vi "PXI-Change AO Gains (gracefully).vi"(0 "Multipliers in":dbl[](array[numeric]), 5 "Gains":dbl[](array[numeric]), 11 "error in (no error)":errorcluster) -> (15 "error out":errorcluster)   [LabVIEW 2015]
uses:
  PXI Globals.vi
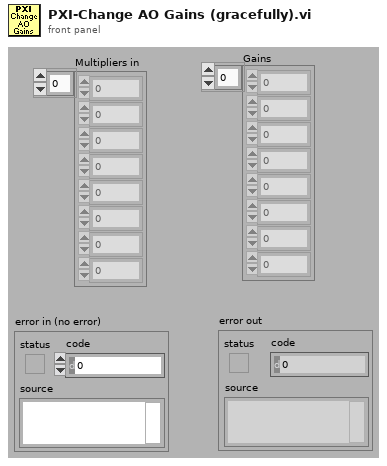
[diagram p1: front panel]
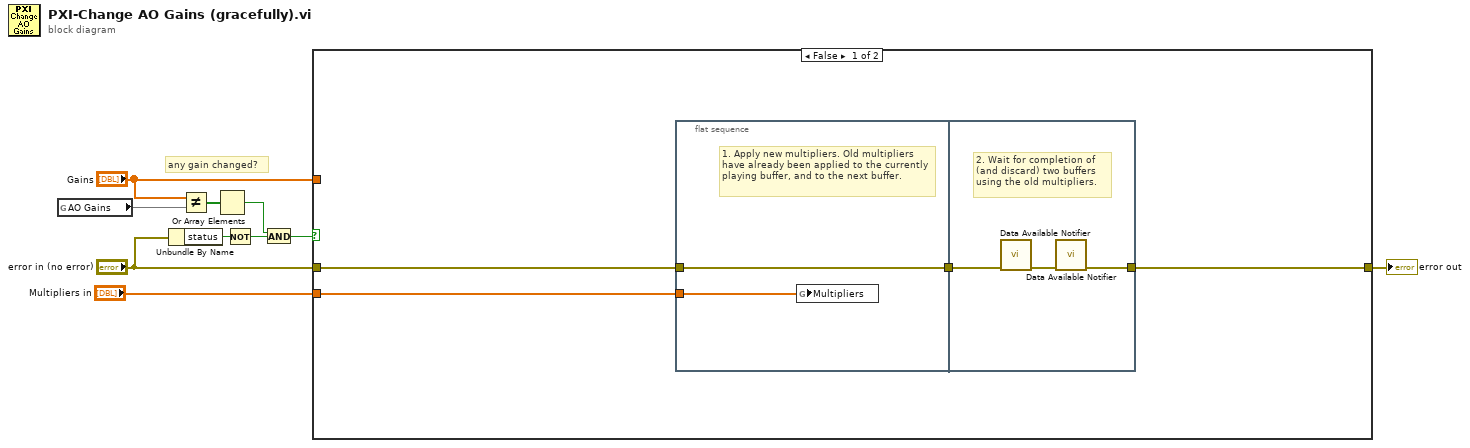
[diagram p0: block diagram]
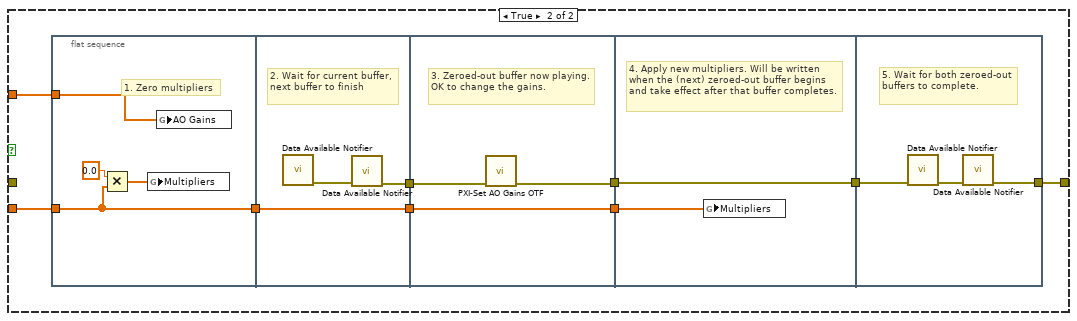
[diagram p2: hidden frame]
diagram:
  # "any gain changed?"
  n1 = global read "PXI Globals.vi" "AO Gains"() -> (w10)
  n2 = Unbundle By Name("error in (no error)") -> ("status"=w9:bool)
  n3 = Not Equal?(x="Gains", y=w10) -> (x != y?=w6:bool[])
  n4 = Or Array Elements(Boolean array=w6) -> (logical OR=w5:bool)
  n5 = Not(x=w9) -> (.not. x?=w8:bool)
  n6 = And(x=w5, y=w8) -> (x .and. y?=w7:bool)
  n7 = case shown="False" w7 {
    tunnel: "error in (no error)" -> [w12 _]
    tunnel: [w11 w28] -> w3
    tunnel: "Multipliers in" -> [w13 w27]
    tunnel: "Gains" -> [_ w20]
    frame False {
      n8 = flat-sequence {
        tunnel: [w15] -> w14
        tunnel: w13 -> [w16]
        tunnel: w12 -> [w15]
        tunnel: [w17] -> w11
        tunnel: w14 -> [w19]
        frame #0 {
          # "1. Apply new multipliers. Old multipliers have already been applied to the currently playing buffer, and to the next buffer."
          n9 = global write "PXI Globals.vi" "Multipliers"(w16) -> ()
        }
        frame #1 {
          # "2. Wait for completion of (and discard) two buffers using the old multipliers."
          n10 = call "Data Available Notifier.vi"("error in (no error)"=w19) -> ("error out"=w18:errorcluster)  [unwired: 12 in, 2 out]
          n11 = call "Data Available Notifier.vi"("error in (no error)"=w18) -> ("error out"=w17:errorcluster)  [unwired: 12 in, 2 out]
        }
      }
    }
    frame True {
      n12 = flat-sequence {
        tunnel: w27 -> [w30]
        tunnel: [w30] -> w25
        tunnel: w20 -> [w29]
        tunnel: [w35] -> w26
        tunnel: w25 -> [w35]
        tunnel: [w33] -> w22
        tunnel: [w37] -> w24
        tunnel: [w36] -> w23
        tunnel: w22 -> [w38]
        tunnel: w26 -> [w36]
        tunnel: w24 -> [w40]
        tunnel: w23 -> [w39]
        tunnel: [w40] -> w21
        tunnel: [w41] -> w28
        tunnel: w21 -> [w43]
        frame #0 {
          # "1. Zero multipliers"
          n13 = Multiply(x=0.0 ("Slide 2"), y=w30) -> (x*y=w31:dbl[])
          n14 = global write "PXI Globals.vi" "Multipliers"(w31) -> ()
          n15 = global write "PXI Globals.vi" "AO Gains"(w29) -> ()
        }
        frame #1 {
          # "2. Wait for current buffer, next buffer to finish"
          n16 = call "Data Available Notifier.vi"() -> ("error out"=w34:errorcluster)  [unwired: 13 in, 2 out]
          n17 = call "Data Available Notifier.vi"("error in (no error)"=w34) -> ("error out"=w33:errorcluster)  [unwired: 12 in, 2 out]
        }
        frame #2 {
          # "3. Zeroed-out buffer now playing. OK to change the gains."
          n18 = call "PXI-Set AO Gains OTF.vi"("error in (no error)"=w38) -> ("error out"=w37:errorcluster)  [unwired: 10 in]
        }
        frame #3 {
          # "4. Apply new multipliers. Will be written when the (next) zeroed-out buffer begins and take effect after that buffer completes."
          n19 = global write "PXI Globals.vi" "Multipliers"(w39) -> ()
        }
        frame #4 {
          # "5. Wait for both zeroed-out buffers to complete."
          n20 = call "Data Available Notifier.vi"("error in (no error)"=w43) -> ("error out"=w42:errorcluster)  [unwired: 12 in, 2 out]
          n21 = call "Data Available Notifier.vi"("error in (no error)"=w42) -> ("error out"=w41:errorcluster)  [unwired: 12 in, 2 out]
        }
      }
    }
  }
  "error out" <- w3
